vi "test_V_exp.vi"() -> ()   [LabVIEW 2017]
panel:
  out "Vini 2":dbl
  out "deltaT":i32
  out "exp(x)":dbl
  out "I Chart":dbl(graph)
  in  "?":dbl=5000.0 format="%#_13g"
  in  "Vo":dbl
  in  "Vini":dbl
  in  "stop":bool
  out "V":dbl
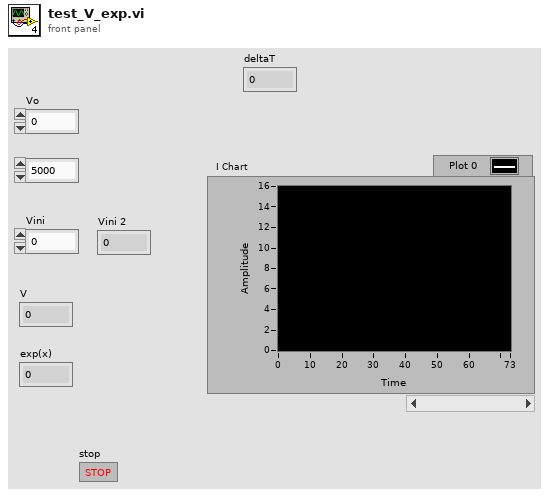
[diagram p1: front panel]
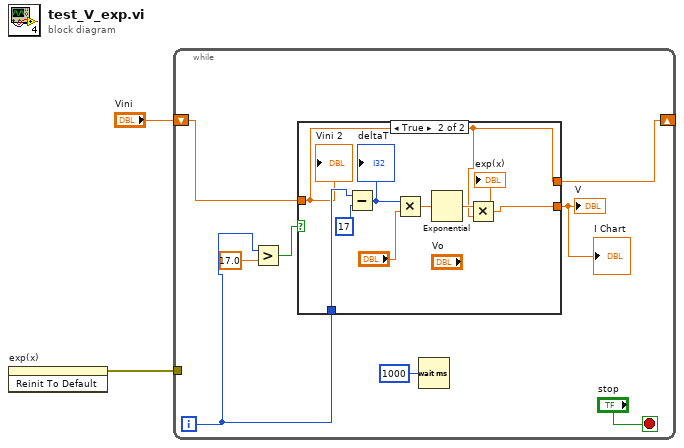
[diagram p0: block diagram]
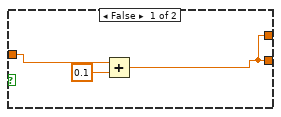
[diagram p2: hidden frame]
diagram:
  n1 = invoke on="exp(x)" class="DigNum (strict)" method="Reinit To Default"() -> (error out=w1:errorcluster)  [unwired: 3 in, 2 out]
  n2 = while {
    shift-right: [w7] -> _
    shift-left: "Vini" -> [w6]
    tunnel: w1 -> [_]
    i -> [w3]
    stop <- "stop" stop-if-true
    n3 = Greater?(x=w3, y=17.0) -> (0:w9:bool)
    n4 = case shown="True" w9 {
      tunnel: w6 -> [w13 w14]
      tunnel: [w11 w14] -> w7
      tunnel: [w11 w18] -> w5
      tunnel: w3 -> [_ w16]
      frame False {
        n5 = Add(x=w13, y=0.1) -> (x+y=w11:dbl)
      }
      frame True {
        n6 = Subtract(x=w16, y=17) -> (x-y=w17:i32)
        "deltaT" <- w17
        n7 = Multiply(x=w17, y="?") -> (x*y=w20:dbl)
        n8 = Exponential(1:w20) -> (0:w19:dbl)
        "exp(x)" <- w19
        n9 = Multiply(x=w19, y=w14) -> (x*y=w18:dbl)
        "Vini 2" <- w14
      }
    }
    "I Chart" <- w5
    "V" <- w5
    n10 = Wait (ms)(milliseconds to wait=u32 1000) -> ()  [unwired: 1 out]
  }
